vi "Trapezoidal Set RPM.vi"(8 "Desired RPM":dbl, 9 "Current RPM":dbl, 11 "Spinning Wheels?":bool) -> (2 "Stage 1 Time":dbl, 3 "RPM":dbl, 5 "Shooter Ready?":bool)   [LabVIEW 2015]
uses:
  Trapezoidal Motion State.ctl
  Common Code/Change Detect Double.vi
  Common Code/Change Detect Boolean.vi
  Robot Code/Robot Global Data.vi
panel:
  out "Current State":T1
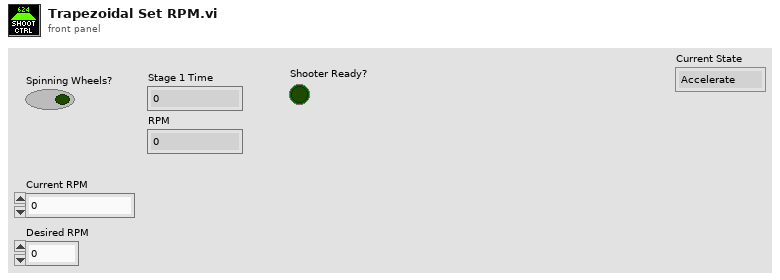
[diagram p1: front panel]
types:
  T1 = typedef "Trapezoidal Motion State.ctl" = enum16{"Accelerate", "Cruise", "Decelerate", "Finish"}
  T2 = typedef "Dashboard Control Data.ctl" = cluster{"Shooter Presets":T3, "Encoder Control":T5, "Steer PID output":cluster{"output high":dbl, "output low":dbl}, " Steer PID gains":cluster{"proportional gain (Kc)":dbl, "integral time (Ti, min)":dbl, "derivative time (Td, min)":dbl}, "Drivetrain Settings":T6, "Vision Packet":T7, "Dashboard Drivetrain Command":T8, "Info/Command Cluster":T10, "Ball Vision Packet":T11, "Intake Presets":T13, "Intake Encoder Control":T15, "Climb Presets":T16, "Ultrasonic Limit":dbl, "Roll Limit":dbl, "Pitch Limit":dbl, "Goal Output Range":cluster{"output high":dbl, "output low":dbl}, "Enabled Systems":T17}
  T3 = typedef "Shooter Presets.ctl" = cluster{"Batter Shot":T4, "Deep Middle Shot":T4, "Manual Shot":T4, "Left Ticks Per Rotation":dbl, "Right Ticks Per Rotation":dbl, "Low Bar Shot":T4, "Shooter RPM Tolerance":dbl, "IIR Filter Power":dbl, "Trigger Power":dbl, "Fire from Load Delay":i32, "Max Angle":dbl, "Min Angle":dbl, "Angle PID gains":cluster{"proportional gain (Kc)":dbl, "integral time (Ti, min)":dbl, "derivative time (Td, min)":dbl}, "Angle Motor Output":cluster{"output high":dbl, "output low":dbl}, "Shooter Angle Tolerance":dbl, "Vision Shoot x^2":dbl, "Vision Shoot x":dbl, "Dist from Axis Cam to Pivot":dbl, "High Goal Center Height":dbl, "Feed Forward Max Accel":dbl, "Feed Forward Kv":dbl, "Backwards Trigger":dbl, "Shot Finish Delay (ms)":dbl, "Angle Max Current":dbl, "Angle Current Trip Time":dbl, "Intake Angle":dbl, "Vision Shoot c":dbl, "Reset?":bool, "Servo Release Delay":dbl, "Servo Idle Angle":i32, "Servo Hold Angle":i32, "Angle Pot x":dbl, "Angle Pot c":dbl, "Ignore Angle?":bool, "Manual Output?":bool, "Manual Out":dbl, "Max RPM":dbl, "Safty Frist Angle":dbl, "Intake Danger Height":dbl, "Angle Pot B":i32, "Angle Pot M":dbl, "FF Finish RPM":dbl}
  T4 = typedef "Shot Presets.ctl" = cluster{"Left Wheel RPM":dbl, "Right Wheel RPM":dbl, "Angle":dbl}
  T5 = typedef "Encoder Control.ctl" = cluster{"Right Tick Constant":dbl, "Left Tick Constant":dbl, "Reset?":bool, "Y Dist":cluster{"PID gains":cluster{"proportional gain (Kc)":dbl, "integral time (Ti, min)":dbl, "derivative time (Td, min)":dbl}}, "Y Stop Thresh":dbl, "Y Stop Speed":dbl}
  T6 = typedef "Drivetrain Settings.ctl" = cluster{"Gyro Tolerance":dbl, "Throttle Ramp (ms)":dbl, "Angular rate compensation":bool, "Throttle to Rate Scale":dbl, "Rate compensation gain":dbl, "Kv":dbl, "Ka":dbl, "Feed Forward P":dbl, "Feed Forward D":dbl, "Goal Vision PID gains":cluster{"proportional gain (Kc)":dbl, "integral time (Ti, min)":dbl, "derivative time (Td, min)":dbl}, "Goal Detection Window":dbl}
  T7 = typedef "Goal Vision Packet.ctl" = cluster{"Distance":dbl, "Center X":dbl, "Center Y":dbl, "Found Target?":bool}
  T8 = typedef "Dashboard Drivetrain Command.ctl" = cluster{"Drivetrain Vision":T9}
  T9 = typedef "Drivetrain Vision.ctl" = cluster{"Goal Window":dbl, "Ball Window":dbl}
  T10 = typedef "Ball Tracking Command Cluster.ctl" = cluster{"Distance to Ball":dbl, "Desired Angle":dbl, "Command":enum16{"Turn to Ball", "Turn to Angle", "Get Distance"}, "Pixels from Center":dbl}
  T11 = typedef "Ball Vision Packet.ctl" = cluster{"Ball Detected?":bool, "Distance to Ball":dbl, "Desired Angle":dbl, "Pixels from Center":dbl, "Tracking mode":T12}
  T12 = typedef "Tracking Mode.ctl" = enum16{"Turn to Ball", "Turn to Angle"}
  T13 = typedef "Intake Presets.ctl" = cluster{"Intake Speed":dbl, "Outake Speed":dbl, "Low Height":dbl, "Half Height":dbl, "Full Height":dbl, "Angle Speed":dbl, "Angle Tolerance":dbl, "Encoder Scale":dbl, "Load Height":dbl, "Output Range":T14, "Rotation Power Max/Min":dbl, "MaxCurrent":dbl, "Intake Trip Time":dbl, "Idle Height":dbl, "Max Height":dbl, "Reset Encoders?":bool, "PID gains":cluster{"proportional gain (Kc)":dbl, "integral time (Ti, min)":dbl, "derivative time (Td, min)":dbl}}
  T14 = typedef "Drivetrain Output Range.ctl" = cluster{"output high":dbl, "output low":dbl}
  T15 = typedef "IntakeEcoderControl.ctl" = cluster{"Arm Tick Constant":dbl, "Reset?":bool, "Y Dist":cluster{"PID gains":cluster{"proportional gain (Kc)":dbl, "integral time (Ti, min)":dbl, "derivative time (Td, min)":dbl}}, "Y Stop Thresh":dbl, "Y Stop Speed":dbl}
  T16 = typedef "Climb Presets.ctl" = cluster{"Pull Power":dbl, "Unpin Power":dbl, "Time to Hold":dbl}
  T17 = typedef "Enabled Systems.ctl" = cluster{"Shoot":bool, "Intake":bool, "DT":bool, "Gyro":bool, "100ms":bool, "US":bool}
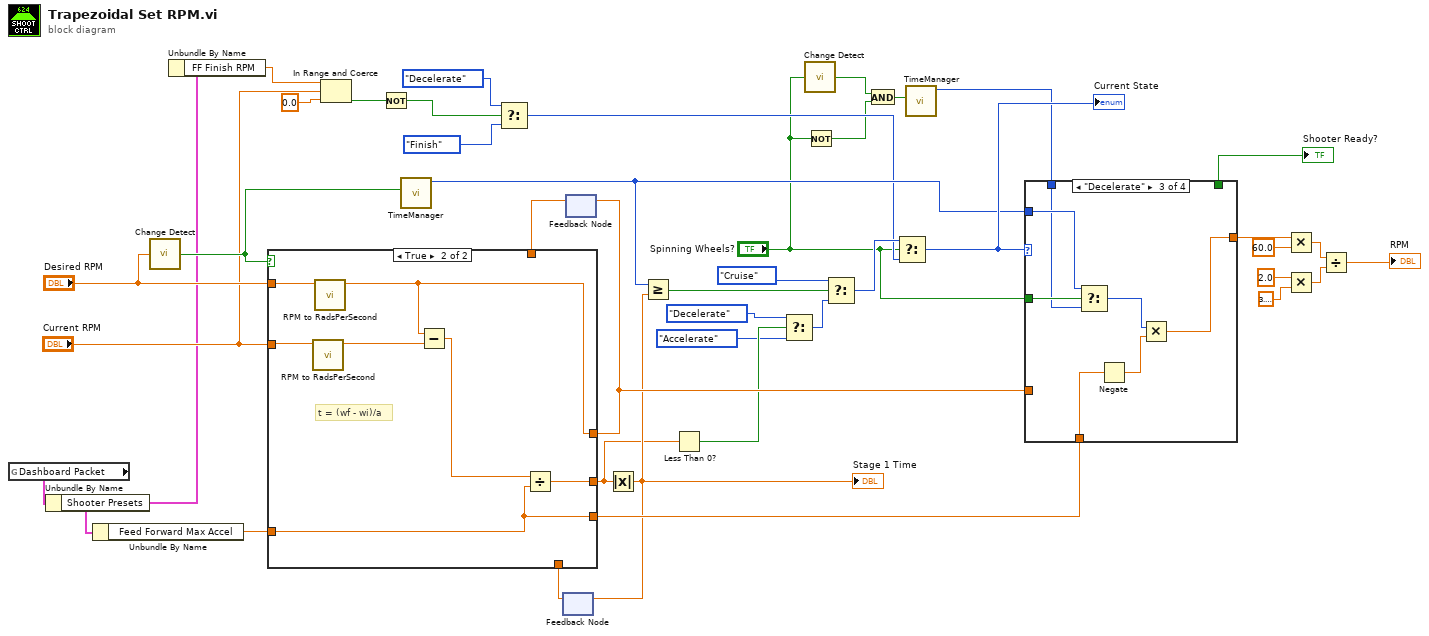
[diagram p0: block diagram]
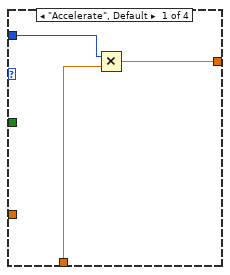
[diagram p2: hidden frame]
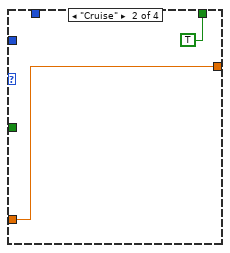
[diagram p3: hidden frame]
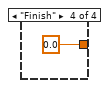
[diagram p4: hidden frame]
diagram:
  n1 = global read "Robot Global Data.vi" "Dashboard Packet"() -> (w24:T2)
  n2 = Unbundle By Name(w24) -> ("Shooter Presets"=w4:T3)
  n3 = Unbundle By Name(w4) -> ("Feed Forward Max Accel"=w23:dbl)
  n4 = call-poly "Change Detect.vi"("In"="Desired RPM") -> ("Changed?"=w7:bool)
  n5 = Unbundle By Name(w4) -> ("FF Finish RPM"=w3:dbl)
  n6 = In Range and Coerce(upper limit=w3, x="Current RPM", lower limit=0.0) -> (In Range?=w2:bool)  [unwired: 1 out]
  n7 = Not(x=w2) -> (.not. x?=w1:bool)
  n8 = call "TimeManager.vi"("Reset?"=w7) -> ("Time Since Reset"=w35:u32)  [unwired: 9 in, 1 out]
  n9 = Select(t=Trapezoidal_Motion_State."Decelerate" ("Enum"), s=w1, f=Trapezoidal_Motion_State."Finish" ("Enum")) -> (s? t:f=w14:T1)
  n10 = feedback #1() -> (w40:dbl)  [unwired: 1 in]
  n11 = feedback #2() -> (w26:dbl)  [unwired: 1 in]
  n12 = case shown="True" w7 {
    tunnel: [w44 w51] -> w21
    tunnel: "Current RPM" -> [_ w48]
    tunnel: "Desired RPM" -> [_ w49]
    tunnel: w40 -> [w44 _]
    tunnel: [w42 w50] -> w34
    tunnel: [w43 w45] -> w25
    tunnel: w26 -> [w43 _]
    tunnel: w23 -> [w42 w50]
    frame False {
    }
    frame True {
      # "t = (wf - wi)/a"
      n13 = call "RPM to RadsPerSecond.vi"("Desired RPM"=w48) -> ("Numeric"=w47:dbl)  [unwired: 10 in]
      n14 = call "RPM to RadsPerSecond.vi"("Desired RPM"=w49) -> ("Numeric"=w45:dbl)  [unwired: 10 in]
      n15 = Subtract(x=w45, y=w47) -> (x-y=w46:dbl)
      n16 = Divide(x=w46, y=w50) -> (x/y=w51:dbl)
    }
  }
  n17 = feedback-in #2(w25) -> ()
  n18 = Absolute Value(x=w21) -> (abs(x)=w22:dbl)
  "Stage 1 Time" <- w22
  n19 = feedback-in #1(w22) -> ()
  n20 = Greater Or Equal?(x=w35, y=w22) -> (x >= y?=w39:bool)
  n21 = Less Than 0?(x=w21) -> (x < 0?=w20:bool)
  n22 = Select(t=Trapezoidal_Motion_State."Decelerate" ("Enum"), s=w20, f=Trapezoidal_Motion_State."Accelerate") -> (s? t:f=w17:T1)
  n23 = call-poly "Change Detect.vi"("In"="Spinning Wheels?") -> ("Changed?"=w13:bool)
  n24 = Not(x="Spinning Wheels?") -> (.not. x?=w12:bool)
  n25 = Select(t=Trapezoidal_Motion_State."Cruise" ("Enum"), s=w39, f=w17) -> (s? t:f=w37:T1)
  n26 = And(x=w13, y=w12) -> (x .and. y?=w11:bool)
  n27 = Select(t=w37, s="Spinning Wheels?", f=w14) -> (s? t:f=w36:T1)
  "Current State" <- w36
  n28 = call "TimeManager.vi"("Reset?"=w11) -> ("Time Since Reset"=w9:u32)  [unwired: 9 in, 1 out]
  n29 = case shown="\"Decelerate\"" w36 {
    tunnel: w35 -> [w54 _ w61 _]
    tunnel: w34 -> [w52 _ w63 _]
    tunnel: [w53 w56 w58 0.0] -> w33
    tunnel: w25 -> [_ w56 _ _]
    tunnel: "Spinning Wheels?" -> [_ _ w62 _]
    tunnel: w9 -> [_ _ w57 _]
    tunnel: [_ TRUE _ _] -> w8
    frame "Accelerate", Default {
      n30 = Multiply(x=w54, y=w52) -> (x*y=w53:dbl)
    }
    frame "Cruise" {
    }
    frame "Decelerate" {
      n31 = Select(t=w61, s=w62, f=w57) -> (s? t:f=w60:u32)
      n32 = Negate(x=w63) -> (-x=w59:dbl)
      n33 = Multiply(x=w60, y=w59) -> (x*y=w58:dbl)
    }
    frame "Finish" {
    }
  }
  "Shooter Ready?" <- w8
  n34 = Multiply(x=w33, y=60.0) -> (x*y=w29:dbl)
  n35 = Multiply(x=2.0, y=3.141592653589793) -> (x*y=w28:dbl)
  n36 = Divide(x=w29, y=w28) -> (x/y=→"RPM":dbl)
